vi "Check Hysteresis_FPGA.vi"(4 "Hysteresis":fxp<+/-,24,7>, 5 "Analog In (Tach)":fxp<+/-,24,7>, 6 "State In":enum16{"Check Hysteresis", "Check Threshold"}(ring), 7 "Threshold":fxp<+/-,24,7>, 8 "Slope":enum16{"falling", "rising"}(ring)) -> (0 "State Out":enum16{"Check Hysteresis", "Check Threshold"}(ring), 1 "Event Ocurred?":bool)   [LabVIEW 2017]
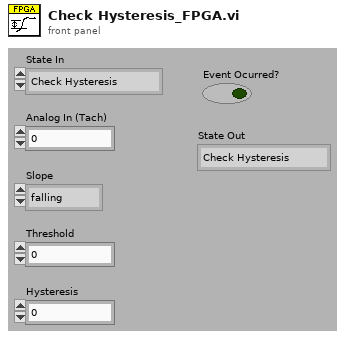
[diagram p1: front panel]
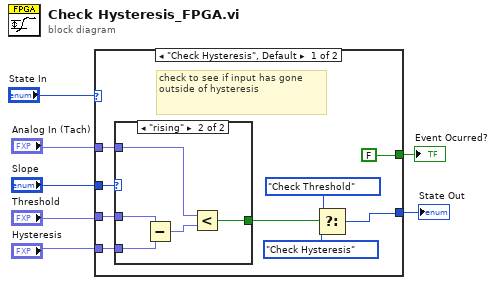
[diagram p0: block diagram]
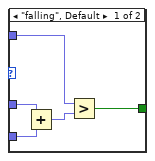
[diagram p2: hidden frame]
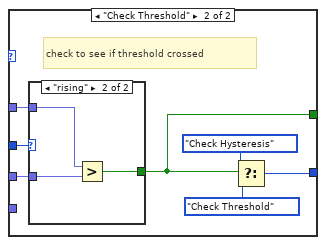
[diagram p3: hidden frame]
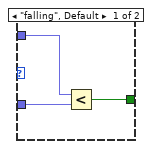
[diagram p4: hidden frame]
diagram:
  n1 = case shown="\"Check Hysteresis\", Default" "State In" {
    tunnel: [w9 w28] -> w6
    tunnel: "Analog In (Tach)" -> [w15 w32]
    tunnel: "Slope" -> [w16 w33]
    tunnel: "Threshold" -> [w14 w31]
    tunnel: "Hysteresis" -> [w13 _]
    tunnel: [FALSE w27] -> w1
    frame "Check Hysteresis", Default {
      # "check to see if input has gone outside of hysteresis"
      n2 = case shown="\"rising\"" w16 {
        tunnel: w15 -> [w19 w23]
        tunnel: w14 -> [w21 w25]
        tunnel: w13 -> [w20 w26]
        tunnel: [w17 w22] -> w12
        frame "falling", Default {
          n3 = Add(x=w21, y=w20) -> (x+y=w18:fxp<+/-,25,8>)
          n4 = Greater?(x=w19, y=w18) -> (0:w17:bool)
        }
        frame "rising" {
          n5 = Subtract(x=w25, y=w26) -> (x-y=w24:fxp<+/-,25,8>)
          n6 = Less?(x=w23, y=w24) -> (x < y?=w22:bool)
        }
      }
      n7 = Select(t=enum16{"Check Hysteresis", "Check Threshold"}."Check Threshold" ("state"), s=w12, f=enum16{"Check Hysteresis", "Check Threshold"}."Check Hysteresis" ("state")) -> (s? t:f=w9:enum16{"Check Hysteresis", "Check Threshold"})
    }
    frame "Check Threshold" {
      # "check to see if threshold crossed"
      n8 = case shown="\"rising\"" w33 {
        tunnel: w32 -> [w36 w39]
        tunnel: w31 -> [w34 w37]
        tunnel: [w35 w38] -> w27
        frame "falling", Default {
          n9 = Less?(x=w36, y=w34) -> (x < y?=w35:bool)
        }
        frame "rising" {
          n10 = Greater?(x=w39, y=w37) -> (0:w38:bool)
        }
      }
      n11 = Select(t=enum16{"Check Hysteresis", "Check Threshold"}."Check Hysteresis" ("state"), s=w27, f=enum16{"Check Hysteresis", "Check Threshold"}."Check Threshold" ("state")) -> (s? t:f=w28:enum16{"Check Hysteresis", "Check Threshold"})
    }
  }
  "State Out" <- w6
  "Event Ocurred?" <- w1
